vi "WPI_HowdyDrive.vi"(8 "error in (no error)":errorcluster, 9 "RightSpeed":dbl, 10 "LeftSpeed":dbl, 11 "RobotDriveDevRef 2":T1={"DevStatus"={"status"=FALSE, "code"=0, "source"=""}, "Motors[]"=[], "Square Inputs"=FALSE, "Max Output"=1.0}) -> (0 "error out":errorcluster, 3 "RobotDriveDevRef":T1={"DevStatus"={"status"=FALSE, "code"=0, "source"=""}, "Motors[]"=[], "Square Inputs"=FALSE, "Max Output"=1.0})   [LabVIEW 2018, in "Drive.lvlib" / "Pod Drive.lvclass"]
doc: "Copy of WPI_RobotDriveMotors.VI\nwe changed the pdm reference to CAN"
uses:
  Pod Drive.lvclass
  <vilib>/Rock Robotics/WPI/RobotDrive/WPI_RobotDriveDevRef.ctl
  <vilib>/Rock Robotics/WPI/MotorControl/WPI_MotorControlDeviceRef.ctl
  <vilib>/Rock Robotics/WPI/MotorControl/WPI_MotorControlType.ctl
  <vilib>/Rock Robotics/SystemInterfaces/DIO/FPGA_DIOPWMChannel.ctl
  <vilib>/Rock Robotics/WPI/PWM/WPI_PWMDeadband.ctl
  <vilib>/Rock Robotics/SystemInterfaces/DIO/FPGA_DIOChannel.ctl
  <vilib>/Rock Robotics/WPI/ThirdParty/Phoenix-LabVIEW/Motor Controller/Controls/CTRE_Phoenix_MotorControl_ControlMode.ctl
  <vilib>/Rock Robotics/WPI/RobotDrive/WPI_RobotDriveSafetyCheck.vi
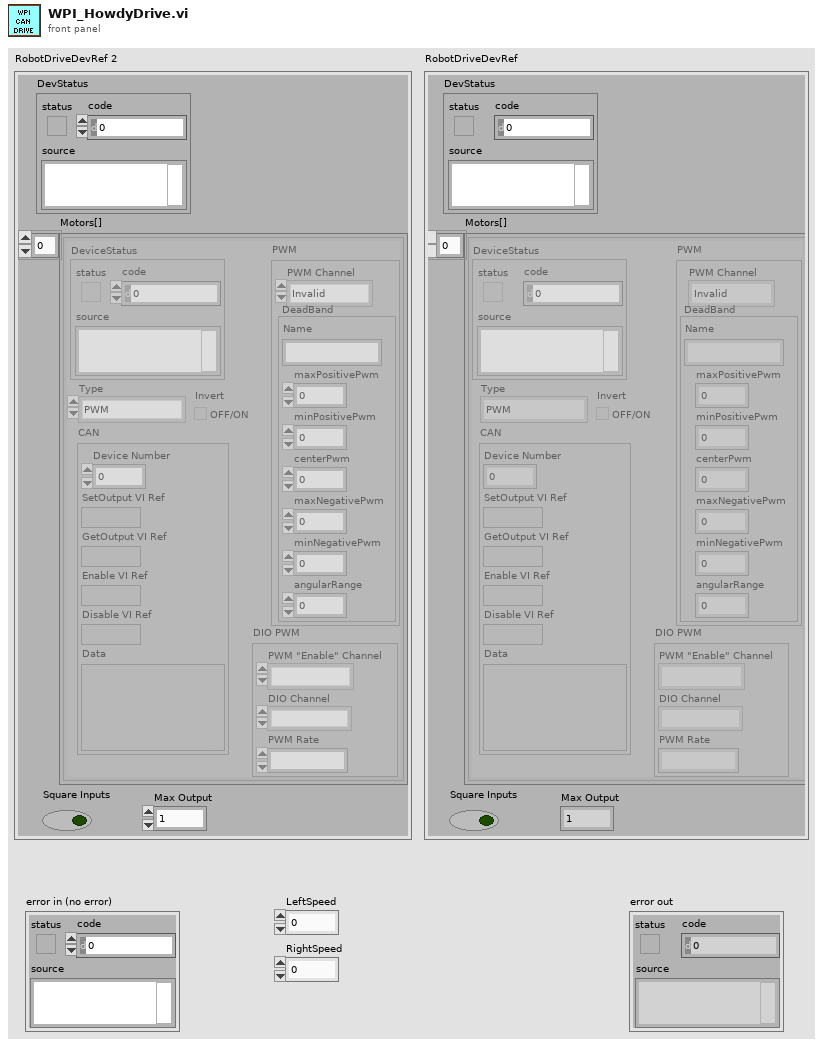
[diagram p1: front panel]
types:
  T1 = typedef "WPI_RobotDriveDevRef.ctl" = cluster{"DevStatus":errorcluster, "Motors[]":T2[], "Square Inputs":bool, "Max Output":dbl}
  T2 = typedef "WPI_MotorControlDeviceRef.ctl" = cluster{"DeviceStatus":errorcluster, "Type":T3, "PWM":cluster{"PWM Channel":T4, "DeadBand":T5}, "CAN":cluster{"Device Number":u8, "SetOutput VI Ref":variant, "GetOutput VI Ref":variant, "Enable VI Ref":variant, "Disable VI Ref":variant, "Data":variant}, "Invert":bool, "DIO PWM":cluster{"PWM \"Enable\" Channel":T4, "DIOChannel":T6, "PWM Rate":dbl}}
  T3 = typedef "WPI_MotorControlType.ctl" = enum16{"PWM", "CAN", "DIO PWM"}
  T4 = typedef "FPGA_DIOPWMChannel.ctl" = enum8{"PWM 0", "PWM 1", "PWM 2", "PWM 3", "PWM 4", "PWM 5", "PWM 6", "PWM 7", "PWM 8", "PWM 9", "PWM MXP 0", "PWM MXP 1", "PWM MXP 2", "PWM MXP 3", "PWM MXP 4", "PWM MXP 5", "PWM MXP 6", "PWM MXP 7", "PWM MXP 8", "PWM MXP 9", "Invalid"}
  T5 = typedef "WPI_PWMDeadband.ctl" = cluster{"Name":string, "maxPositivePwm":i32, "minPositivePwm":i32, "centerPwm":i32, "maxNegativePwm":i32, "minNegativePwm":i32, "angularRange":u16}
  T6 = typedef "FPGA_DIOChannel.ctl" = enum8{"DIO 0", "DIO 1", "DIO 2", "DIO 3", "DIO 4", "DIO 5", "DIO 6", "DIO 7", "DIO 8", "DIO 9", "DIO MXP 0", "DIO MXP 1", "DIO MXP 2", "DIO MXP 3", "DIO MXP 4", "DIO MXP 5", "DIO MXP 6", "DIO MXP 7", "DIO MXP 8", "DIO MXP 9", "DIO MXP 10", "DIO MXP 11", "DIO MXP 12", "DIO MXP 13", "DIO MXP 14", "DIO MXP 15", "SPI Port CS1", "SPI Port CS2", "SPI Port CS3", "SPI Port MISO", "SPI Port MOSI", "Invalid"}
  T7 = typedef "CTRE_Phoenix_MotorControl_ControlMode.ctl" = u16
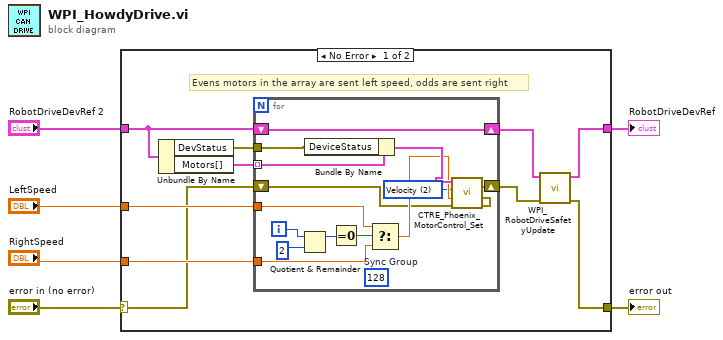
[diagram p0: block diagram]
diagram:
  n1 = case shown="No Error" "error in (no error)" {
    selector: "error in (no error)" -> [w7 w32]
    tunnel: "RobotDriveDevRef 2" -> [w10 w31]
    tunnel: [w15 w31] -> w5
    tunnel: "LeftSpeed" -> [w14 _]
    tunnel: "RightSpeed" -> [w13 _]
    tunnel: [w16 w32] -> w1
    frame No Error {
      # "Evens motors in the array are sent left speed, odds are sent right"
      n2 = Unbundle By Name(w10) -> ("DevStatus"=w8:errorcluster, "Motors[]"=w9:T2[])
      n3 = for {
        tunnel: w14 -> [w26]
        tunnel: w13 -> [w25]
        shift-right: [w17] -> w12
        shift-left: w7 -> [w18]
        shift-right: [w24] -> w11
        shift-left: w10 -> [w24]
        tunnel: w9 -> [w22] mode=indexing
        tunnel: w8 -> [w23]
        i -> [w29]
        w19 = T7 2 items=["PercentOutput"=0, "Position"=1, "Velocity"=2, "Current"=3, "Follower"=5, "MotionProfile"=6, "MotionMagic"=7, "MotionProfileArc"=10, "Disabled"=15] ("Control Mode")
        (unwired) u8 128  # Sync Group
        n4 = Quotient & Remainder(x=w29, y=2) -> (x-y*floor(x/y)=w28:i32)  [unwired: 1 out]
        n5 = Bundle By Name(cluster=w22, "DeviceStatus"=w23) -> (w21:T2)
        n6 = Equal To 0?(x=w28) -> (x = 0?=w27:bool)
        n7 = Select(t=w26, s=w27, f=w25) -> (s? t:f=w20:dbl)
        n8 = call <vilib>:"CTRE_Phoenix_MotorControl_Set.vi"("error in (no error)"=w18, "Output"=w20, "Control Mode"=w19, "PhoenixMotorControlDevRef"=w21) -> ("error out"=w17:errorcluster)  [unwired: 6 in, 1 out]
      }
      n9 = call <vilib>:"WPI_RobotDriveSafetyUpdate.vi"("error in (no error)"=w12, "RobotDriveDevRef"=w11) -> ("error out"=w16:errorcluster, "RobotDriveDevRef"=w15:T1)  [unwired: 8 out]
    }
    frame Error {
    }
  }
  "RobotDriveDevRef" <- w5
  "error out" <- w1
